vi "Builtins.vi"(6 "args":string[](array[string]), 7 "QD Plugins Dir":path, 8 "error in (no error)":errorcluster, 9 "Shift?":bool, 10 "Focus":enum8{"FP", "BD"}(ring), 11 "VI Refnum":refnum<vi>) -> (0 "error out":errorcluster)   [LabVIEW 2019]
doc: "Built-in script shortcuts\n\nUsage: Ctrl-Space + \"<shortcut>\" + Ctrl-S\n\nCreated by: Ryan Pacini\n\n[SCRIPT]\n--=Rename Label\n--c=Rename Caption\n--iconlib=Edit Library Icon\n0=Open in File Explore\na=Arrange\naa=Align Left Edges\nad=Align Right Edges\nah=Align Horizontal Centers\nas=Align Bottom Edges\nav=Align Vertical Centers\naw=Align Top Edges\nc=Connect Pane\ncf=Cluster Size Fit\nch=Cluster Size Horizontally\ncn=Cluster Size None\ncv=Cluster Size Vertically\nd=Distribute Vertical Compress\nda=Distribute Left Edges\ndd=Distribute Right Edges\ndf=Distribute Horizontal Compress \ndh=Distribute Horizontal Centers\ndhg=Distribute Horizontal Gap\nds=Distribute Bottom Edges\ndv=Distribute Vertical Centers\ndvg=Distribute Vertical Gap\ndw=Distribute Top Edges\ne=Resizes Window\ner=Error Structure\nhb=Hide Inc/Dec Buttons\nhc=Hide Caption\nhi=Hide Index Display\nhl=Hide Label\nhr=Hide Radix\nhs=Hide Scrollbars\nm=Merge Icon Layers\no=Reset Panel Origins\nrb=Radix Binary or Backslash\nrd=Radix Decimal or Normal\nrx=Radix Hex\nsb=Show Inc/Dec Buttons\nsc=Show Caption\nsi=Show Index Display\nsl=Show Label\nss=Show Scrollbars\nsel=Select Controls and Indicators\nselc=Select Controls\nseli=Select Indicators\nseln=Select None\nsg=Snap to Panel Grid\nu8=Change to U8\nu16=Change to U16\nu32=Change to U32\nu64=Change to U64\ni8=Change to I8\ni16=Change to I16\ni32=Change to I32\ni64=Change to I64\nsgl=Change to SGL\ndbl=Change to DBL\next=Change to EXT\ncsg=Change to CSG\ncdb=Change to CDB\ncxt=Change to CXT"
uses:
  _Builtins/Align.ctl
  _Builtins/Distribute.ctl
  _Builtins/Selection.ctl
  _Builtins/Builtins.lvlib
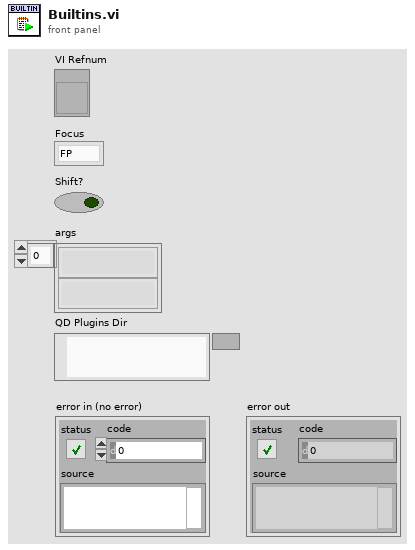
[diagram p1: front panel]
types:
  T1 = typedef "Builtins.lvlib/Align.ctl" = enum8{"Top Edges", "Vertical Centers", "Bottom Edges", "Left Edges", "Horizontal Centers", "Right Edges"}
  T2 = enum32{"Extended Precision", "Double Precision", "Single Precision", "Long", "Word", "Byte", "Unsigned Long", "Unsigned Word", "Unsigned Byte", "Complex Extended", "Complex Double", "Complex Single", "Quad", "Unsigned Quad", "Fixed-Point"}
  T3 = enum8{"None", "SizeToFit", "Horizontally", "Vertically"}
  T4 = typedef "Builtins.lvlib/Distribute.ctl" = enum8{"Top Edges", "Vertical Centers", "Bottom Edges", "Vertical Gap", "Vertical Compress", "Left Edges", "Horizontal Centers", "Right Edges", "Horizontal Gap", "Horizontal Compress"}
  T5 = typedef "Builtins.lvlib/Selection.ctl" = enum8{"None", "Controls", "Indicators", "Both"}
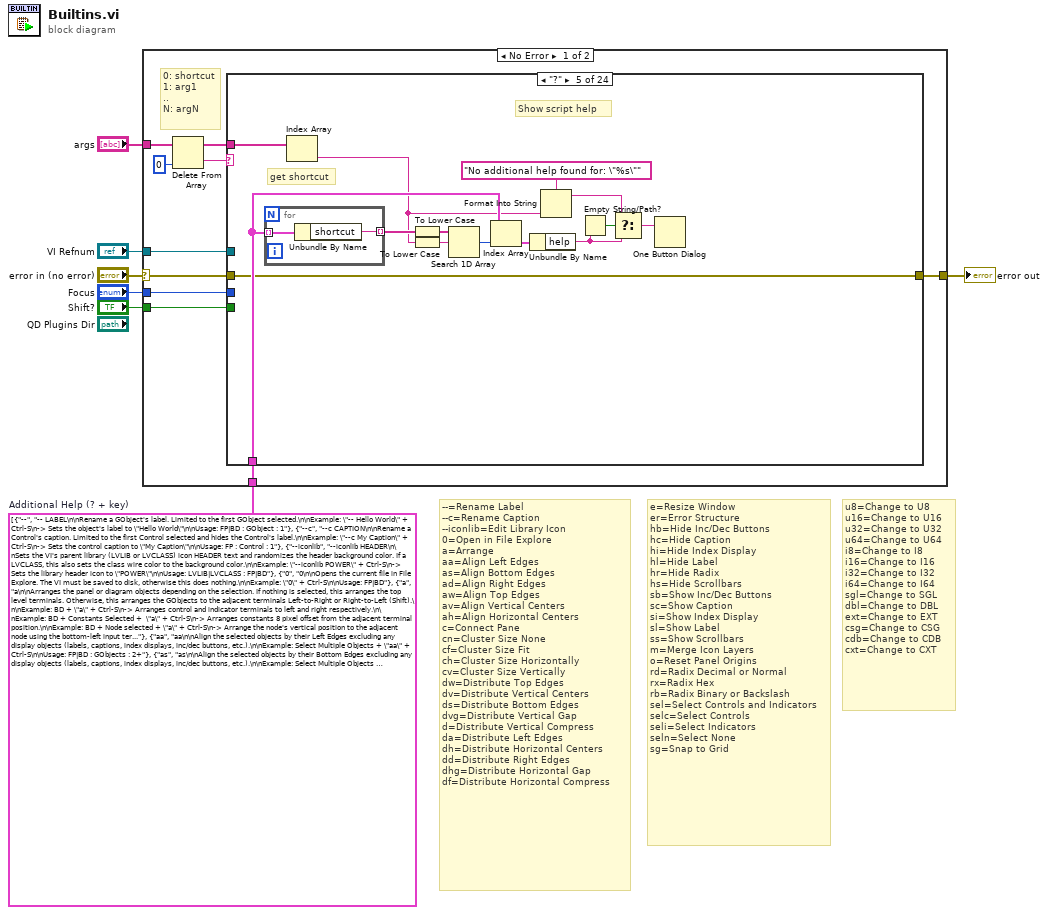
[diagram p0: block diagram]
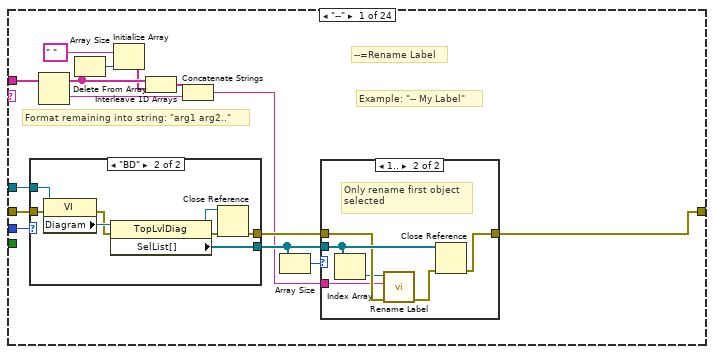
[diagram p2: hidden frame]
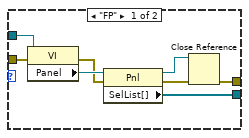
[diagram p3: hidden frame]
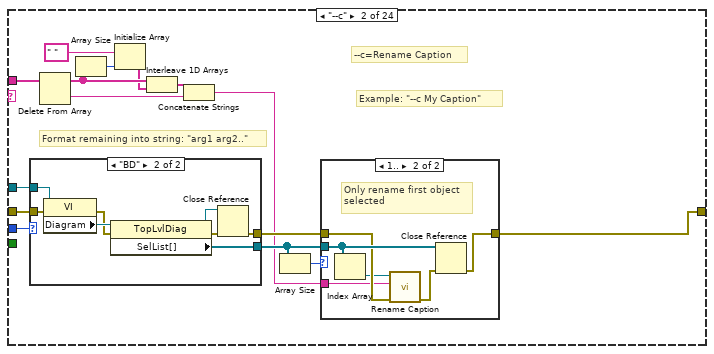
[diagram p5: hidden frame]
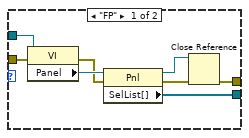
[diagram p6: hidden frame]
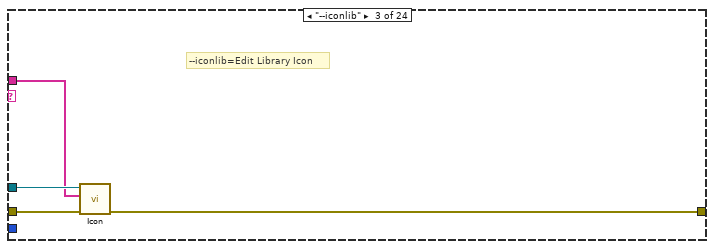
[diagram p8: hidden frame]
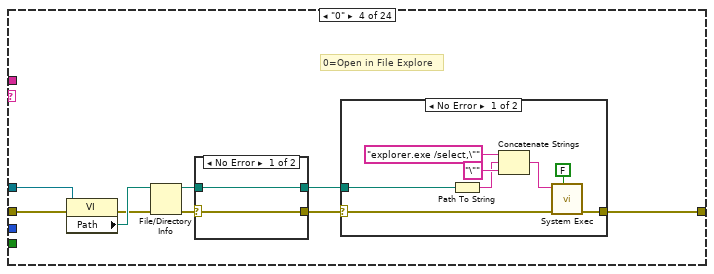
[diagram p9: hidden frame]
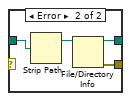
[diagram p10: hidden frame]
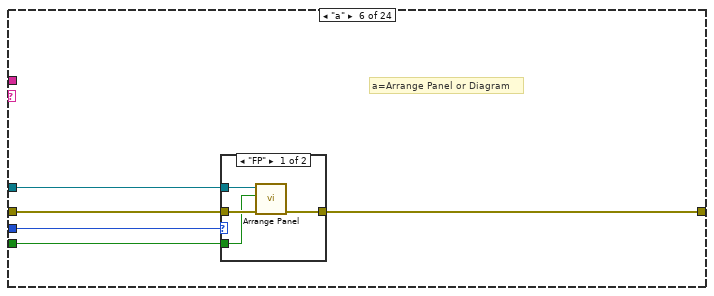
[diagram p12: hidden frame]
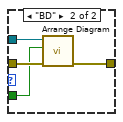
[diagram p13: hidden frame]
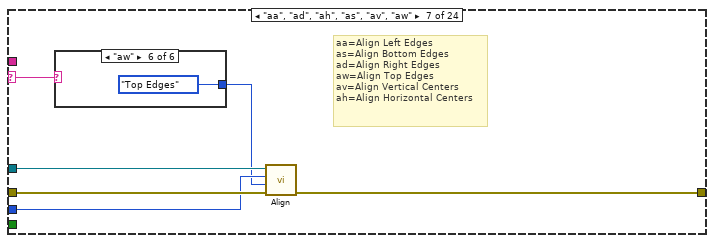
[diagram p14: hidden frame]
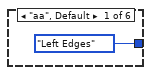
[diagram p15: hidden frame]
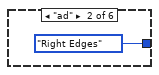
[diagram p16: hidden frame]
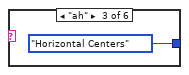
[diagram p17: hidden frame]
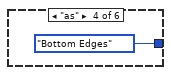
[diagram p18: hidden frame]
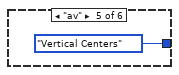
[diagram p19: hidden frame]
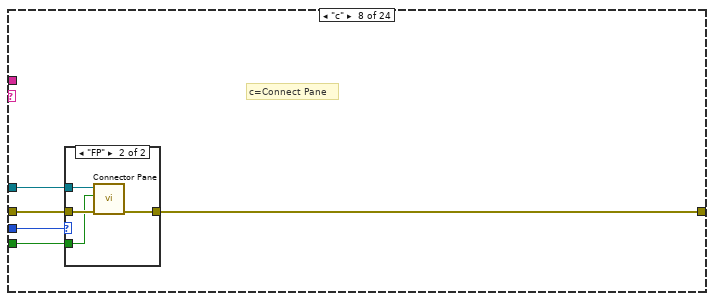
[diagram p20: hidden frame]
diagram:
  w1 = cluster{"shortcut":string, "help":string}[] [{"shortcut"="--", "help"="-- LABEL\n\nRename a GObject's label. Limited to the first GObject selected.\n\nExample: \"-- Hello World\" + Ctrl-S\n-> Sets the object's label to \"Hello World\"\n\nUsage: FP|BD : GObject : 1"}, {"shortcut"="--c", "help"="--c CAPTION\n\nRename a Control's caption. Limited to the first Control selected and hides the Control's label.\n\nExample: \"--c My Caption\" + Ctrl-S\n-> Sets the control caption to \"My Caption\"\n\nUsage: FP : Control : 1"}, {"shortcut"="--iconlib", "help"="--iconlib HEADER\n\nSets the VI's parent library (LVLIB or LVCLASS) icon HEADER text and randomizes the header background color. If a LVCLASS, this also sets the class wire color to the background color.\n\nExample: \"--iconlib POWER\" + Ctrl-S\n-> Sets the library header icon to \"POWER\"\n\nUsage: LVLIB|LVCLASS : FP|BD"}, {"shortcut"="0", "help"="0\n\nOpens the current file in File Explore. The VI must be saved to disk, otherwise this does nothing.\n\nExample: \"0\" + Ctrl-S\n\nUsage: FP|BD"}, {"shortcut"="a", "help"="a\n\nArranges the panel or diagram objects depending on the selection. If nothing is selected, this arranges the top level terminals. Otherwise, this arranges the GObjects to the adjacent terminals Left-to-Right or Right-to-Left (Shift).\n\nExample: BD + \"a\" + Ctrl-S\n-> Arranges control and indicator terminals to left and right respectively.\n\nExample: BD + Constants Selected +  \"a\" + Ctrl-S\n-> Arranges constants 8 pixel offset from the adjacent terminal position.\n\nExample: BD + Node selected + \"a\" + Ctrl-S\n-> Arrange the node's vertical position to the adjacent node using the bottom-left input terminal.\n\nExample: BD + Node selected + \"a\" + Ctrl-Shift-S\n-> Arrange the node's vertical position to the adjacent node using the bottom-right output terminal.\n\nUsage: FP|BD : GObjects : 0+"}, {"shortcut"="aa", "help"="aa\n\nAlign the selected objects by their Left Edges excluding any display objects (labels, captions, index displays, inc/dec buttons, etc.).\n\nExample: Select Multiple Objects + \"aa\" + Ctrl-S\n\nUsage: FP|BD : GObjects : 2+"}, {"shortcut"="as", "help"="as\n\nAlign the selected objects by their Bottom Edges excluding any display objects (labels, captions, index displays, inc/dec buttons, etc.).\n\nExample: Select Multiple Objects + \"as\" + Ctrl-S\n\nUsage: FP|BD : GObjects : 2+"}, {"shortcut"="ad", "help"="ad\n\nAlign the selected objects by their Right Edges excluding any display objects (labels, captions, index displays, inc/dec buttons, etc.).\n\nExample: Select Multiple Objects + \"ad\" + Ctrl-S\n\nUsage: FP|BD : GObjects : 2+"}, {"shortcut"="aw", "help"="aw\n\nAlign the selected objects by their Top Edges excluding any display objects (labels, captions, index displays, inc/dec buttons, etc.).\n\nExample: Select Multiple Objects + \"aw\" + Ctrl-S\n\nUsage: FP|BD : GObjects : 2+"}, {"shortcut"="av", "help"="av\n\nAlign the selected objects by their Vertical Centers excluding any display objects (labels, captions, index displays, inc/dec buttons, etc.).\n\nExample: Select Multiple Objects + \"av\" + Ctrl-S\n\nUsage: FP|BD : GObjects : 2+"}, {"shortcut"="ah", "help"="ah\n\nAlign the selected objects by their Horizontal Centers excluding any display objects (labels, captions, index displays, inc/dec buttons, etc.).\n\nExample: Select Multiple Objects + \"ah\" + Ctrl-S\n\nUsage: FP|BD : GObjects : 2+"}, {"shortcut"="c", "help"="c\n\nWire the Front Panel Controls to the VI Conntector Pane in order of position (top-left to bottom-right). If nothing is selected all unwired controls are connected. Error clusters are wired to the bottom-left and bottom-right terminal. Hold Shift to start wiring by inner columns. Wired terminals are skipped.\n\nExample: FP + \"c\" + Ctrl-S\n-> Wire all controls to VI Connector Pane.\n\nExample: FP + Select Control + \"c\" + Ctrl-Shift-S\n-> Wire selected control to VI Connecto Pane starting with inner column.\n\nUsage: FP : Controls : 0+"}, {"shortcut"="cn", "help"="cn\n\nAutosize the Cluster to None.\n\nExample: Select Cluster + \"cn\" + Ctrl-S\n\nUsage: FP|BD : Cluster : 1+"}, {"shortcut"="cv", "help"="cv\n\nAutosize the Cluster Vertically.\n\nExample: Select Cluster + \"cv\" + Ctrl-S\n\nUsage: FP|BD : Cluster : 1+"}, {"shortcut"="ch", "help"="ch\n\nAutosize the Cluster Horizontally.\n\nExample: Select Cluster + \"ch\" + Ctrl-S\n\nUsage: FP|BD : Cluster : 1+"}, {"shortcut"="cf", "help"="cf\n\nAutosize the Cluster to Fit.\n\nExample: Select Cluster + \"cf\" + Ctrl-S\n\nUsage: FP|BD : Cluster : 1+"}, {"shortcut"="dw", "help"="dw\n\nDistibute the selected objects by their Top Edges including any display objects (labels, captions, index display, inc/dec buttons, etc.).\n\nExample: Select Multiple Objects + \"dw\" + Ctrl-S\n\nUsage: FP|BD : GObjects : 2+"}, {"shortcut"="dv", "help"="dv\n\nDistibute the selected objects by their Vertical Centers including any display objects (labels, captions, index display, inc/dec buttons, etc.).\n\nExample: Select Multiple Objects + \"dv\" + Ctrl-S\n\nUsage: FP|BD : GObjects : 2+"}, {"shortcut"="ds", "help"="ds\n\nDistibute the selected objects by their Bottom Edges including any display objects (labels, captions, index display, inc/dec buttons, etc.).\n\nExample: Select Multiple Objects + \"ds\" + Ctrl-S\n\nUsage: FP|BD : GObjects : 2+"}, {"shortcut"="dvg", "help"="dvg\n\nDistibute the selected objects by their Vertical Gap including any display objects (labels, captions, index display, inc/dec buttons, etc.).\n\nExample: Select Multiple Objects + \"dvg\" + Ctrl-S\n\nUsage: FP|BD : GObjects : 2+"}, {"shortcut"="d", "help"="d\n\nDistibute the selected objects by their Vertical Compress including any display objects (labels, captions, index display, inc/dec buttons, etc.).\n\nExample: Select Multiple Objects + \"d\" + Ctrl-S\n\nUsage: FP|BD : GObjects : 2+"}, {"shortcut"="da", "help"="da\n\nDistibute the selected objects by their Left Edges including any display objects (labels, captions, index display, inc/dec buttons, etc.).\n\nExample: Select Multiple Objects + \"da\" + Ctrl-S"}, {"shortcut"="dh", "help"="dh\n\nDistibute the selected objects by their Horizontal Centers including any display objects (labels, captions, index display, inc/dec buttons, etc.).\n\nExample: Select Multiple Objects + \"dh\" + Ctrl-S\n\nUsage: FP|BD : GObjects : 2+"}, {"shortcut"="dd", "help"="dd\n\nDistibute the selected objects by their Right Edges including any display objects (labels, captions, index display, inc/dec buttons, etc.).\n\nExample: Select Multiple Objects + \"dd\" + Ctrl-S\n\nUsage: FP|BD : GObjects : 2+"}, {"shortcut"="dhg", "help"="dhg\n\nDistibute the selected objects by their Horizontal Gap including any display objects (labels, captions, index display, inc/dec buttons, etc.).\n\nExample: Select Multiple Objects + \"dhg\" + Ctrl-S\n\nUsage: FP|BD : GObjects : 2+"}, {"shortcut"="df", "help"="df\n\nDistibute the selected objects by their Horizontal Compress including any display objects (labels, captions, index display, inc/dec buttons, etc.).\n\nExample: Select Multiple Objects + \"df\" + Ctrl-S\n\nUsage: FP|BD : GObjects : 2+"}, {"shortcut"="e", "help"="e\n\nResize the panel or diagram window to content. This resets the front panel origins to zero.\n\nExample: BD + \"e\" + Ctrl-S\n-> Resizes the diagram window to content with padding.\n\nExample: FP + \"e\" + Ctrl-S\n-> Resets the panel origins and resizes window to bottom-right padding.\n\nUsage: FP|BD"}, {"shortcut"="er", "help"="er\n\nOn the diagram, this wires the selected case structure to the error in and error out terminals. If the case structure selector is already wired, this does nothing. On the panel, this replaces the selected controls with the Error In 3D controls. \n\nExample: BD + Case Structure with Error wires + \"er\" + Ctrl-S\n-> Wires the error terminals to case structure.\n\nExample: FP + Select Control + \"er\" + Ctrl-S\n-> Replaces control with Error In 3D ctl.\n\nUsage: BD : Case Structure : 1 | FP : Control : 1"}, {"shortcut"="hb", "help"="hb\n\nHide the selected Control's Increment/Decrement buttons.\n\nExample: Select Numeric Control + \"hb\" + Ctrl-S\n\nUsage: FP : Controls : 1+"}, {"shortcut"="hc", "help"="hc\n\nHide the selected control's Caption.\n\nExample: Select Control + \"hc\" + Ctrl-S\n\nUsage: FP : Controls : 1+"}, {"shortcut"="hi", "help"="hi\n\nHide the selected array object's Index Display.\n\nExample: Select Array + \"hi\" + Ctrl-S\n\nUsage: FP|BD : Array : 1+"}, {"shortcut"="hl", "help"="hl\n\nHide the selected GObject's Label.\n\nExample: Select GObject + \"hl\" + Ctrl-S\n\nUsage: FP|BD : GObjects : 1+"}, {"shortcut"="hr", "help"="hr\n\nHide the selected Numeric or String Radix Display.\n\nExample: Select Object + \"hr\" + Ctrl-S\n\nUsage: FP|BD : Numeric|String | 1+"}, {"shortcut"="hs", "help"="hs\n\nHide the selected String or Container Vertical Scrollbar.\n\nExample: Select String + \"hs\" + Ctrl-S\n\nUsage: FP|BD : String|Container : 1+"}, {"shortcut"="sb", "help"="sb\n\nShow the selected Control's Increment/Decrement Buttons.\n\nExample: Select Numeric Control + \"sb\" + Ctrl-S\n\nUsage: FP : Controls : 1+"}, {"shortcut"="sc", "help"="sc\n\nShow the selected Control's Caption. This uses the controls label if the caption is not defined.\n\nExample: Select Control + \"sc\" + Ctrl-S\n\nUsage: FP : Controls : 1+"}, {"shortcut"="si", "help"="si\n\nShow the selected Array's Index Display.\n\nExample: Select Array + \"si\" + Ctrl-S\n\nUsage: FP|BD : Array : 1+"}, {"shortcut"="sl", "help"="sl\n\nShow the selected GObject's Label.\n\nExample: Select GObject + \"sl\" + Ctrl-S\n\nUsage: FP|BD : GObjects : 1+"}, {"shortcut"="ss", "help"="ss\n\nShow the selected String or Container Vertical Scrollbars.\n\nExample: Select String + \"ss\" + Ctrl-S\n\nUsage: FP|BD : String|Container | 1+"}, {"shortcut"="m", "help"="m\n\nMerge VI Icon Layers to reduce memory and avoid icon template conflicts.\n\nExample: \"m\" + Ctrl-S\n\nUsage: FP|BD"}, {"shortcut"="o", "help"="o\n\nReset all Front Panel Origins to (0, 0).\n\nExample: \"o\" + Ctrl-S\n\nUsage: FP"}, {"shortcut"="rd", "help"="rd\n\nShow the selected Numeric or String Radix in Decimal (or Default Text).\n\nExample: Select Numeric Control + \"rd\" + Ctrl-S\n-> Shows the radix in decimal (%d)\n\nExample: Select String Control + \"rd\" + Ctrl-S\n-> Shows the radix in default text\n\nUsage: FP|BD : Numeric|String : 1+"}, {"shortcut"="rx", "help"="rx\n\nShow the selected Numeric or String Radix in Hex. If a numeric, this will pad the hex with zeros depending on the numeric representation.\n\nExample: Select U16 Numeric Control + \"rx\" + Ctrl-S\n-> Shows the radix in hex (%04x = '0x0000')\n\nExample: Select String Control + \"rx\" + Ctrl-S\n-> Shows the radix in hex text\n\nUsage: FP|BD : Numeric|String : 1+"}, {"shortcut"="rb", "help"="rb\n\nShow the selected Numeric or String Radix in Binary (or Backslash). If a numeric, this will pad the binary with zeros depending on the numeric representation.\n\nExample: Select U8 Numeric Control + \"rb\" + Ctrl-S\n-> Shows the radix in binary (%08b = '0b00000000')\n\nExample: Select String Control + \"rb\" + Ctrl-S\n-> Shows the radix in backslash text\n\nUsage: FP|BD : Numeric|String : 1+"}, {"shortcut"="sel", "help"="sel\n\nSelect all top-level Control and Indicator Terminals. Used to chain multiple scripts together.\n\nExample: FP + \"sel\" + Ctrl-S\n-> Selects all controls and indicators.\n\nExample: BD + \"sel\" + Ctrl-S\n-> Selects all control and indicator terminals on the top-level diagram.\n\nUsage: FP|BD"}, {"shortcut"="selc", "help"="selc\n\nSelect all top-level Control Terminals. Used to chain multiple scripts together.\n\nExample: FP + \"selc\" + Ctrl-S\n-> Selects all controls.\n\nExample: BD + \"selc\" + Ctrl-S\n-> Selects all control terminals on the top-level diagram.\n\nUsage: FP|BD"}, {"shortcut"="seli", "help"="seli\n\nSelect all top-level Indicator Terminals. Used to chain multiple scripts together.\n\nExample: FP + \"seli\" + Ctrl-S\n-> Selects all indicators.\n\nExample: BD + \"seli\" + Ctrl-S\n-> Selects all indicator terminals on the top-level diagram.\n\nUsage: FP|BD"}, {"shortcut"="seln", "help"="seln\n\nDe-select all. Used to chain multiple scripts together.\n\nExample: FP + \"selc\" + Ctrl-S\n-> De-selects all.\n\nExample: BD + \"selc\" + Ctrl-S\n-> De-selects all.\n\nUsage: FP|BD"}, {"shortcut"="sg", "help"="sg\n\nSnap the selected controls to the nearest panel grid position. If nothing is selected, this snaps all controls. Default grid size is 12 px.\n\nExample: FP + \"sg\" + Ctrl-S\n-> Snaps all controls to nearest grid position.\n\nUsage: FP : Controls : 0+"}, {"shortcut"="u8", "help"="u8\n\nChanges the Numeric Representation to U8.\n\nExample: Select Numeric + \"u8\" + Ctrl-S\n\nUsage: FP|BD : Numeric : 1+"}, {"shortcut"="u16", "help"="u16\n\nChanges the Numeric Representation to U16.\n\nExample: Select Numeric + \"u16\" + Ctrl-S\n\nUsage: FP|BD : Numeric : 1+"}, {"shortcut"="u32", "help"="u32\n\nChanges the Numeric Representation to U32.\n\nExample: Select Numeric + \"u32\" + Ctrl-S\n\nUsage: FP|BD : Numeric : 1+"}, {"shortcut"="u64", "help"="u64\n\nChanges the Numeric Representation to U64.\n\nExample: Select Numeric + \"u64\" + Ctrl-S\n\nUsage: FP|BD : Numeric : 1+"}, {"shortcut"="i8", "help"="i8\n\nChanges the Numeric Representation to I8.\n\nExample: Select Numeric + \"i8\" + Ctrl-S\n\nUsage: FP|BD : Numeric : 1+"}, {"shortcut"="i16", "help"="i16\n\nChanges the Numeric Representation to I16.\n\nExample: Select Numeric + \"i16\" + Ctrl-S\n\nUsage: FP|BD : Numeric : 1+"}, {"shortcut"="i32", "help"="i32\n\nChanges the Numeric Representation to I32.\n\nExample: Select Numeric + \"i32\" + Ctrl-S\n\nUsage: FP|BD : Numeric : 1+"}, {"shortcut"="i64", "help"="i64\n\nChanges the Numeric Representation to I64.\n\nExample: Select Numeric + \"i64\" + Ctrl-S\n\nUsage: FP|BD : Numeric : 1+"}, {"shortcut"="sgl", "help"="sgl\n\nChanges the Numeric Representation to SGL.\n\nExample: Select Numeric + \"sgl\" + Ctrl-S\n\nUsage: FP|BD : Numeric : 1+"}, {"shortcut"="dbl", "help"="dbl\n\nChanges the Numeric Representation to DBL.\n\nExample: Select Numeric + \"dbl\" + Ctrl-S\n\nUsage: FP|BD : Numeric : 1+"}, {"shortcut"="ext", "help"="ext\n\nChanges the Numeric Representation to EXT.\n\nExample: Select Numeric + \"ext\" + Ctrl-S\n\nUsage: FP|BD : Numeric : 1+"}, {"shortcut"="csg", "help"="csg\n\nChanges the Numeric Representation to CSG.\n\nExample: Select Numeric + \"csg\" + Ctrl-S\n\nUsage: FP|BD : Numeric : 1+"}, {"shortcut"="cdb", "help"="cdb\n\nChanges the Numeric Representation to CDB.\n\nExample: Select Numeric + \"cdb\" + Ctrl-S\n\nUsage: FP|BD : Numeric : 1+"}, {"shortcut"="cxt", "help"="cxt\n\nChanges the Numeric Representation to CXT.\n\nExample: Select Numeric + \"cxt\" + Ctrl-S\n\nUsage: FP|BD : Numeric : 1+"}]  # Additional Help (? + key)
  # "u8=Change to U8\nu16=Change to U16\nu32=Change to U32\nu64=Change to U64\ni8=Change to I8\ni16=Change to I16\ni32=Change to I32\ni64=Change to I64\nsgl=Change to SGL\ndbl=Change to DBL\next=Change to EXT\ncsg=Change to CSG\ncdb=Change to CDB\ncxt=Change to CXT"
  # "e=Resize Window\ner=Error Structure\nhb=Hide Inc/Dec Buttons\nhc=Hide Caption\nhi=Hide Index Display\nhl=Hide Label\nhr=Hide Radix\nhs=Hide Scrollbars\nsb=Show Inc/Dec Buttons\nsc=Show Caption\nsi=Show Index Display\nsl=Show Label\nss=Show Scrollbars\nm=Merge Icon Layers\no=Reset Panel Origins\nrd=Radix Decimal or Normal\nrx=Radix Hex\nrb=Radix Binary or Backslash\nsel=Select Controls and Indicators\nselc=Select Controls\nseli=Select Indicators\nseln=Select None\nsg=Snap to Grid"
  # "--=Rename Label\n--c=Rename Caption\n--iconlib=Edit Library Icon\n0=Open in File Explore\na=Arrange\naa=Align Left Edges\nas=Align Bottom Edges\nad=Align Right Edges\naw=Align Top Edges\nav=Align Vertical Centers\nah=Align Horizontal Centers\nc=Connect Pane\ncn=Cluster Size None\ncf=Cluster Size Fit\nch=Cluster Size Horizontally\ncv=Cluster Size Vertically\ndw=Distribute Top Edges\ndv=Distribute Vertical Centers\nds=Distribute Bottom Edges\ndvg=Distribute Vertical Gap\nd=Distribute Vertical Compress\nda=Distribute Left Edges\ndh=Distribute Horizontal Centers\ndd=Distribute Right Edges\ndhg=Distribute Horizontal Gap\ndf=Distribute Horizontal Compress"
  n1 = case shown="No Error" "error in (no error)" {
    selector: "error in (no error)" -> [w17 w384]
    tunnel: "VI Refnum" -> [w16 _]
    tunnel: "Focus" -> [w15 _]
    tunnel: "Shift?" -> [w13 _]
    tunnel: "args" -> [w12 _]
    tunnel: [w14 w384] -> w2
    tunnel: w1 -> [w8 _]
    frame No Error {
      # "0: shortcut\n1: arg1\n..\nN: argN"
      n2 = Delete From Array(array=w12, index=0) -> (deleted portion=w11:string, array with subset deleted=w10:string[])  [unwired: 1 in]
      n3 = case shown="\"?\"" w11 {
        selector: w11 -> [_ _ _ _ _ _ w151 _ w177 w231 w241 _ _ w271 w286 w300 w314 w327 w343 _ _ w363 _ w382]
        tunnel: w17 -> [w32 w70 w97 w106 w128 w142 w156 w167 w176 w230 w246 w259 w264 w270 w284 w298 w312 w326 w342 w352 w356 w367 w375 w383]
        tunnel: w16 -> [w31 w69 w96 w105 _ w141 w155 w166 w175 w229 w245 w260 w263 w269 w283 w297 w311 w325 w341 w353 w357 w366 w374 _]
        tunnel: w15 -> [w26 w64 _ _ _ w139 w153 w164 w173 w228 w244 w257 w261 w268 w282 w296 w310 w324 w340 _ w354 w364 w372 _]
        tunnel: [w29 w67 w95 w104 w128 w140 w154 w165 w174 w225 w243 w258 w262 w265 w280 w293 w307 w321 w337 w351 w355 w365 w373 w383] -> w14
        tunnel: w13 -> [_ _ _ _ _ w138 _ w163 _ _ _ _ _ _ _ _ _ _ _ _ _ _ _ _]
        tunnel: w10 -> [w19 w57 w94 _ w133 _ _ _ _ _ _ _ _ _ _ _ _ _ _ _ _ _ _ _]
        tunnel: w8 -> [_ _ _ _ w130 _ _ _ _ _ _ _ _ _ _ _ _ _ _ _ _ _ _ _]
        frame "--" {
          # "Example: \"-- My Label\""
          # "Format remaining into string: \"arg1 arg2..\""
          # "--=Rename Label"
          n4 = case shown="\"BD\"" w26 {
            tunnel: w32 -> [w40 w48]
            tunnel: w31 -> [w39 w47]
            tunnel: [w35 w43] -> w30
            tunnel: [w33 w41] -> w27
            frame "FP" {
              n5 = property class="VI"(reference=w39, error in=w40) -> (error out=w37:errorcluster, "Panel"=w38:refnum<vi>)  [unwired: 1 out]
              n6 = property class="Pnl"(reference=w38, error in=w37) -> (reference out=w36:refnum<vi>, error out=w34:errorcluster, "SelList[]"=w35:refnum<vi>[])
              n7 = Close Reference(reference=w36, error in (no error)=w34) -> (error out=w33:errorcluster)
            }
            frame "BD" {
              n8 = property class="VI"(reference=w47, error in=w48) -> (error out=w45:errorcluster, "Diagram"=w46:refnum<vi>)  [unwired: 1 out]
              n9 = property class="TopLvlDiag"(reference=w46, error in=w45) -> (reference out=w44:refnum<vi>, error out=w42:errorcluster, "SelList[]"=w43:refnum<vi>[])
              n10 = Close Reference(reference=w44, error in (no error)=w42) -> (error out=w41:errorcluster)
            }
          }
          n11 = Delete From Array(array=w19) -> (deleted portion=w20:string, array with subset deleted=w22:string[])  [unwired: 2 in]
          n12 = Array Size(array=w22) -> (size(s)=w24:i32)
          n13 = Initialize Array(" ", w24) -> (w21:string[])
          n14 = Interleave 1D Arrays(w22, w21) -> (w25:string[])
          n15 = Concatenate Strings(w25, w20) -> (w18:string)
          n16 = Array Size(array=w30) -> (size(s)=w28:i32)
          n17 = case shown="1.." w28 {
            tunnel: w27 -> [w49 w53]
            tunnel: w30 -> [_ w55]
            tunnel: w18 -> [_ w50]
            tunnel: [w49 w54] -> w29
            frame ..0 {
              # "Nothing selected"
            }
            frame 1.. {
              # "Only rename first object\nselected"
              n18 = Index Array(array=w55) -> (element=w52:refnum<vi>)  [unwired: 1 in]
              n19 = call "Rename Label.vi"("error in (no error)"=w53, "Label"=w50, "GObject in"=w52) -> ("error out"=w51:errorcluster)  [unwired: 6 in, 2 out]
              n20 = Close Reference(reference=w55, error in (no error)=w51) -> (error out=w54:errorcluster)
            }
          }
        }
        frame "--c" {
          # "Example: \"--c My Caption\""
          # "Format remaining into string: \"arg1 arg2..\""
          # "--c=Rename Caption"
          n21 = case shown="\"BD\"" w64 {
            tunnel: w70 -> [w78 w86]
            tunnel: w69 -> [w77 w85]
            tunnel: [w73 w81] -> w68
            tunnel: [w71 w79] -> w65
            frame "FP" {
              n22 = property class="VI"(reference=w77, error in=w78) -> (error out=w75:errorcluster, "Panel"=w76:refnum<vi>)  [unwired: 1 out]
              n23 = property class="Pnl"(reference=w76, error in=w75) -> (reference out=w74:refnum<vi>, error out=w72:errorcluster, "SelList[]"=w73:refnum<vi>[])
              n24 = Close Reference(reference=w74, error in (no error)=w72) -> (error out=w71:errorcluster)
            }
            frame "BD" {
              n25 = property class="VI"(reference=w85, error in=w86) -> (error out=w83:errorcluster, "Diagram"=w84:refnum<vi>)  [unwired: 1 out]
              n26 = property class="TopLvlDiag"(reference=w84, error in=w83) -> (reference out=w82:refnum<vi>, error out=w80:errorcluster, "SelList[]"=w81:refnum<vi>[])
              n27 = Close Reference(reference=w82, error in (no error)=w80) -> (error out=w79:errorcluster)
            }
          }
          n28 = Delete From Array(array=w57) -> (deleted portion=w58:string, array with subset deleted=w60:string[])  [unwired: 2 in]
          n29 = Array Size(array=w60) -> (size(s)=w62:i32)
          n30 = Initialize Array(" ", w62) -> (w59:string[])
          n31 = Interleave 1D Arrays(w60, w59) -> (w63:string[])
          n32 = Concatenate Strings(w63, w58) -> (w56:string)
          n33 = Array Size(array=w68) -> (size(s)=w66:i32)
          n34 = case shown="1.." w66 {
            tunnel: w65 -> [w87 w91]
            tunnel: w68 -> [_ w93]
            tunnel: w56 -> [_ w89]
            tunnel: [w87 w92] -> w67
            frame ..0 {
              # "Nothing selected"
            }
            frame 1.. {
              # "Only rename first object\nselected"
              n35 = Index Array(array=w93) -> (element=w90:refnum<vi>)  [unwired: 1 in]
              n36 = call "Rename Caption.vi"("error in (no error)"=w91, "Caption"=w89, "GObject in"=w90) -> ("error out"=w88:errorcluster)  [unwired: 6 in, 2 out]
              n37 = Close Reference(reference=w93, error in (no error)=w88) -> (error out=w92:errorcluster)
            }
          }
        }
        frame "--iconlib" {
          # "--iconlib=Edit Library Icon"
          n38 = call "Icon.vi"("error in (no error)"=w97, "Args"=w94, "VI Refnum in"=w96) -> ("error out"=w95:errorcluster)  [unwired: 7 in, 1 out]
        }
        frame "0" {
          # "0=Open in File Explore"
          n39 = property class="VI"(reference=w105, error in=w106) -> (error out=w98:errorcluster, "Path"=w103:path)  [unwired: 1 out]
          n40 = File/Directory Info(path=w103, error in=w98) -> (path out=w102:path, error out=w100:errorcluster)  [unwired: 5 out]
          n41 = case shown="No Error" w100 {
            selector: w100 -> [w107 _]
            tunnel: w102 -> [w108 w112]
            tunnel: [w107 w110] -> w101
            tunnel: [w108 w109] -> w99
            frame No Error {
            }
            frame Error {
              n42 = Strip Path(path=w112) -> (stripped path=w111:path)  [unwired: 1 out]
              n43 = File/Directory Info(path=w111) -> (path out=w109:path, error out=w110:errorcluster)  [unwired: 1 in, 5 out]
            }
          }
          n44 = case shown="No Error" w101 {
            selector: w101 -> [w113 w121]
            tunnel: [w115 w121] -> w104
            tunnel: w99 -> [w114 _]
            frame No Error {
              n45 = Path To String(path=w114) -> (string=w116:string)
              n46 = Concatenate Strings("explorer.exe /select,\"" ("string"), w116, "\"" ("string")) -> (w118:string)
              n47 = call <vilib>:"System Exec.vi"("wait until completion? (T)"=FALSE, "error in (no error)"=w113, "command line"=w118) -> ("error out"=w115:errorcluster)  [unwired: 5 in, 3 out]
            }
            frame Error {
            }
          }
        }
        frame "?" {
          # "Show script help"
          # "get shortcut"
          n48 = for {
            tunnel: w130 -> [w137] mode=indexing
            tunnel: [w136] -> w135 mode=indexing
            n49 = Unbundle By Name(w137) -> ("shortcut"=w136:string)
          }
          n50 = Index Array(array=w133) -> (element=w124:string)  [unwired: 1 in]
          n51 = To Lower Case(string=w135) -> (all lower case string=w134:string[])
          n52 = To Lower Case(string=w124) -> (all lower case string=w132:string)
          n53 = Search 1D Array(1D array=w134, element=w132) -> (index of element=w131:i32)  [unwired: 1 in]
          n54 = Index Array(array=w130, index=w131) -> (element=w129:cluster{"shortcut":string, "help":string})
          n55 = Unbundle By Name(w129) -> ("help"=w126:string)
          n56 = Format Into String(format string="No additional help found for: \"%s\"", w124) -> (resulting string=w122:string)  [unwired: 2 in, 1 out]
          n57 = Empty String/Path?(string/path=w126) -> (empty?=w127:bool)
          n58 = Select(t=w122, s=w127, f=w126) -> (s? t:f=w125:string)
          n59 = One Button Dialog(message=w125) -> ()  [unwired: 1 in, 1 out]
        }
        frame "a" {
          # "a=Arrange Panel or Diagram"
          n60 = case shown="\"FP\"" w139 {
            tunnel: w142 -> [w146 w150]
            tunnel: w141 -> [w145 w149]
            tunnel: w138 -> [w144 w148]
            tunnel: [w143 w147] -> w140
            frame "FP" {
              n61 = call "Arrange Panel.vi"("error in (no error)"=w146, "Shift?"=w144, "VI Refnum in"=w145) -> ("error out"=w143:errorcluster)  [unwired: 7 in, 1 out]
            }
            frame "BD" {
              n62 = call "Arrange Diagram.vi"("error in (no error)"=w150, "Shift?"=w148, "VI Refnum in"=w149) -> ("error out"=w147:errorcluster)  [unwired: 7 in, 1 out]
            }
          }
        }
        frame "aa", "ad", "ah", "as", "av", "aw" {
          # "aa=Align Left Edges\nas=Align Bottom Edges\nad=Align Right Edges\naw=Align Top Edges\nav=Align Vertical Centers\nah=Align Horizontal Centers"
          n63 = case shown="\"aw\"" w151 {
            tunnel: [Align."Left Edges" ("Align Type") Align."Right Edges" ("Align Type") Align."Horizontal Centers" ("Align Type") Align."Bottom Edges" ("Align Type") Align."Vertical Centers" ("Align Type") Align."Top Edges" ("Align Type")] -> w152
            frame "aa", Default {
            }
            frame "ad" {
            }
            frame "ah" {
            }
            frame "as" {
            }
            frame "av" {
            }
            frame "aw" {
            }
          }
          n64 = call "Align.vi"("error in (no error)"=w156, "Align Type"=w152, "Panel"=w153, "VI Refnum in"=w155) -> ("error out"=w154:errorcluster)  [unwired: 6 in, 1 out]
        }
        frame "c" {
          # "c=Connect Pane"
          n65 = case shown="\"FP\"" w164 {
            tunnel: w167 -> [w168 w172]
            tunnel: w166 -> [_ w171]
            tunnel: [w168 w170] -> w165
            tunnel: w163 -> [_ w169]
            frame "BD" {
            }
            frame "FP" {
              n66 = call "Connector Pane.vi"("error in (no error)"=w172, "Wire Middle? (F)"=w169, "VI Refnum in"=w171) -> ("error out"=w170:errorcluster)  [unwired: 7 in, 1 out]
            }
          }
        }
        frame "cdb", "csg", "cxt", "dbl", "ext", "i16", "i32", "i64", "i8", "sgl", "u16", "u32", "u64", "u8" {
          # "**WARNING: Changing Representation clears the panel/diagram Selection List (LV2019 bug)"
          # "sgl=Change to SGL\ndbl=Change to DBL\next=Change to EXT\ncsg=Change to CSG\ncdb=Change to CDB\ncxt=Change to CXT"
          # "u8=Change to U8\nu16=Change to U16\nu32=Change to U32\nu64=Change to U64\ni8=Change to I8\ni16=Change to I16\ni32=Change to I32\ni64=Change to I64"
          n67 = case shown="\"i16\"" w177 {
            tunnel: [T2."Unsigned Byte" ("Representation") T2."Unsigned Word" ("Representation") T2."Unsigned Long" ("Representation") T2."Unsigned Quad" ("Representation") T2."Byte" ("Representation") T2."Word" ("Representation") T2."Long" ("Representation") T2."Quad" ("Representation") T2."Single Precision" ("Representation") T2."Double Precision" ("Representation") T2."Extended Precision" ("Representation") T2."Complex Single" ("Representation") T2."Complex Double" ("Representation") T2."Complex Extended" ("Representation")] -> w178
            frame "u8", Default {
            }
            frame "u16" {
            }
            frame "u32" {
            }
            frame "u64" {
            }
            frame "i8" {
            }
            frame "i16" {
            }
            frame "i32" {
            }
            frame "i64" {
            }
            frame "sgl" {
            }
            frame "dbl" {
            }
            frame "ext" {
            }
            frame "csg" {
            }
            frame "cdb" {
            }
            frame "cxt" {
            }
          }
          n68 = case shown="\"BD\"" w173 {
            tunnel: w178 -> [w190 w206]
            tunnel: w176 -> [w187 w203]
            tunnel: w175 -> [w186 w202]
            tunnel: [w180 w196] -> w174
            frame "BD" {
              n69 = property class="VI"(reference=w186, error in=w187) -> (error out=w188:errorcluster, "Diagram"=w189:refnum<vi>)  [unwired: 1 out]
              n70 = property class="TopLvlDiag"(reference=w189, error in=w188) -> (reference out=w184:refnum<vi>, error out=w185:errorcluster, "SelList[]"=w183:refnum<vi>[])
              n71 = for {
                tunnel: w183 -> [w194] mode=indexing
                tunnel: w190 -> [w193]
                shift-right: [w191] -> w182
                shift-left: w185 -> [w192]
                n72 = call "Numeric Representation.vi"("error in (no error)"=w192, "Representation"=w193, "GObject in"=w194) -> ("error out"=w191:errorcluster)  [unwired: 6 in, 2 out]
              }
              n73 = invoke class="TopLvlDiag" method="Make Selection"(reference=w184, error in=w182, "Objects"=w183) -> (reference out=w179:refnum<vi>, error out=w181:errorcluster)  [unwired: 1 in, 2 out]
              n74 = Close Reference(reference=w179, error in (no error)=w181) -> (error out=w180:errorcluster)
            }
            frame "FP" {
              n75 = property class="VI"(reference=w202, error in=w203) -> (error out=w204:errorcluster, "Panel"=w205:refnum<vi>)  [unwired: 1 out]
              n76 = property class="Pnl"(reference=w205, error in=w204) -> (reference out=w200:refnum<vi>, error out=w201:errorcluster, "SelList[]"=w199:refnum<vi>[])
              n77 = for {
                tunnel: w199 -> [w210] mode=indexing
                tunnel: w206 -> [w209]
                shift-right: [w207] -> w198
                shift-left: w201 -> [w208]
                n78 = call "Numeric Representation.vi"("error in (no error)"=w208, "Representation"=w209, "GObject in"=w210) -> ("error out"=w207:errorcluster)  [unwired: 6 in, 2 out]
              }
              n79 = invoke class="Pnl" method="Make Selection"(reference=w200, error in=w198, "Objects"=w199) -> (reference out=w195:refnum<vi>, error out=w197:errorcluster)  [unwired: 1 in, 2 out]
              n80 = Close Reference(reference=w195, error in (no error)=w197) -> (error out=w196:errorcluster)
            }
          }
        }
        frame "cf", "ch", "cn", "cv" {
          # "cn=Cluster Size None\ncf=Cluster Size Fit\nch=Cluster Size Horizontally\ncv=Cluster Size Vertically"
          n81 = case shown="\"cf\"" w231 {
            tunnel: [T3."SizeToFit" ("AutoSize") T3."Horizontally" ("AutoSize") T3."None" ("AutoSize") T3."Vertically" ("AutoSize")] -> w232
            frame "cf" {
            }
            frame "ch" {
            }
            frame "cn" {
            }
            frame "cv", Default {
            }
          }
          n82 = call "Selection List.vi"("error in (no error)"=w230, "Focus"=w228, "VI Refnum in"=w229) -> ("error out"=w227:errorcluster, "SelList[]"=w226:refnum<vi>[])  [unwired: 5 in, 2 out]
          n83 = for {
            tunnel: w226 -> [w234] mode=indexing
            tunnel: w232 -> [w233]
            shift-right: [w235] -> w225
            shift-left: w227 -> [w236]
            n84 = call "Cluster Autosize.vi"("error in (no error)"=w236, "AutoSize"=w233, "GObject in"=w234) -> ("error out"=w235:errorcluster)  [unwired: 6 in, 2 out]
          }
        }
        frame "d", "da", "dd", "df", "dh", "dhg", "ds", "dv", "dvg", "dw" {
          # "dw=Distribute Top Edges\ndv=Distribute Vertical Centers\nds=Distribute Bottom Edges\ndvg=Distribute Vertical Gap\nd=Distribute Vertical Compress\nda=Distribute Left Edges\ndh=Distribute Horizontal Centers\ndd=Distribute Right Edges\ndhg=Distribute Horizontal Gap\ndf=Distribute Horizontal Compress"
          n85 = case shown="\"d\", Default" w241 {
            tunnel: [Distribute."Vertical Compress" ("Distribute Type") Distribute."Left Edges" ("Distribute Type") Distribute."Right Edges" ("Distribute Type") Distribute."Horizontal Compress" ("Distribute Type") Distribute."Horizontal Centers" ("Distribute Type") Distribute."Horizontal Gap" ("Distribute Type") Distribute."Bottom Edges" ("Distribute Type") Distribute."Vertical Centers" ("Distribute Type") Distribute."Vertical Gap" ("Distribute Type") Distribute."Top Edges" ("Distribute Type")] -> w242
            frame "d", Default {
            }
            frame "da" {
            }
            frame "dd" {
            }
            frame "df" {
            }
            frame "dh" {
            }
            frame "dhg" {
            }
            frame "ds" {
            }
            frame "dv" {
            }
            frame "dvg" {
            }
            frame "dw" {
            }
          }
          n86 = call "Distribute.vi"("error in (no error)"=w246, "Distribute Type"=w242, "Panel"=w244, "VI Refnum in"=w245) -> ("error out"=w243:errorcluster)  [unwired: 6 in, 1 out]
        }
        frame "e" {
          # "e=Resize Window"
          n87 = call "Resize Window.vi"("error in (no error)"=w259, "Focus"=w257, "VI Refnum in"=w260) -> ("error out"=w258:errorcluster)  [unwired: 7 in, 1 out]
        }
        frame "er" {
          # "er=Error Structure"
          n88 = call "Error Structure.vi"("error in (no error)"=w264, "Focus"=w261, "VI Refnum in"=w263) -> ("error out"=w262:errorcluster)  [unwired: 7 in, 1 out]
        }
        frame "hb", "sb" {
          # "hb=Hide Inc/Dec Buttons\nsb=Show Inc/Dec Buttons"
          n89 = case shown="\"sb\"" w271 {
            tunnel: [enum8{"hide", "show"}."hide" ("inc/dec") enum8{"hide", "show"}."show" ("inc/dec")] -> w272
            frame "hb", Default {
            }
            frame "sb" {
            }
          }
          n90 = call "Selection List.vi"("error in (no error)"=w270, "Focus"=w268, "VI Refnum in"=w269) -> ("error out"=w267:errorcluster, "SelList[]"=w266:refnum<vi>[])  [unwired: 5 in, 2 out]
          n91 = for {
            tunnel: w266 -> [w276] mode=indexing
            tunnel: w272 -> [w273]
            shift-right: [w274] -> w265
            shift-left: w267 -> [w275]
            n92 = call "Visible IncDec.vi"("error in (no error)"=w275, "inc/dec"=w273, "GObject in"=w276) -> ("error out"=w274:errorcluster)  [unwired: 5 in, 3 out]
          }
        }
        frame "hc", "sc" {
          # "hc=Hide Caption\nsc=Show Caption"
          n93 = case shown="\"sc\", Default" w286 {
            tunnel: [enum8{"hide", "show"}."hide" ("label") enum8{"hide", "show"}."show" ("label")] -> w285
            frame "hc" {
            }
            frame "sc", Default {
            }
          }
          n94 = call "Selection List.vi"("error in (no error)"=w284, "Focus"=w282, "VI Refnum in"=w283) -> ("error out"=w281:errorcluster, "SelList[]"=w279:refnum<vi>[])  [unwired: 5 in, 2 out]
          n95 = for {
            tunnel: w279 -> [w290] mode=indexing
            shift-right: [w289] -> w280
            shift-left: w281 -> [w288]
            tunnel: w285 -> [w287]
            n96 = call "Visible Caption.vi"("error in (no error)"=w288, "caption"=w287, "GObject in"=w290) -> ("error out"=w289:errorcluster)  [unwired: 5 in, 3 out]
          }
        }
        frame "hi", "si" {
          # "hi=Hide Index Display\nsi=Show Index Display"
          n97 = case shown="\"si\", Default" w300 {
            tunnel: [enum8{"hide", "show"}."hide" ("label") enum8{"hide", "show"}."show" ("label")] -> w299
            frame "hi" {
            }
            frame "si", Default {
            }
          }
          n98 = call "Selection List.vi"("error in (no error)"=w298, "Focus"=w296, "VI Refnum in"=w297) -> ("error out"=w295:errorcluster, "SelList[]"=w294:refnum<vi>[])  [unwired: 5 in, 2 out]
          n99 = for {
            tunnel: w294 -> [w304] mode=indexing
            shift-right: [w301] -> w293
            shift-left: w295 -> [w302]
            tunnel: w299 -> [w303]
            n100 = call "Visible Index.vi"("error in (no error)"=w302, "index display"=w303, "GObject in"=w304) -> ("error out"=w301:errorcluster)  [unwired: 5 in, 3 out]
          }
        }
        frame "hl", "sl" {
          # "hl=Hide Label\nsl=Show Label"
          n101 = case shown="\"hl\"" w314 {
            tunnel: [enum8{"hide", "show"}."hide" ("label") enum8{"hide", "show"}."show" ("label")] -> w313
            frame "hl" {
            }
            frame "sl", Default {
            }
          }
          n102 = call "Selection List.vi"("error in (no error)"=w312, "Focus"=w310, "VI Refnum in"=w311) -> ("error out"=w309:errorcluster, "SelList[]"=w308:refnum<vi>[])  [unwired: 5 in, 2 out]
          n103 = for {
            tunnel: w308 -> [w318] mode=indexing
            shift-right: [w317] -> w307
            shift-left: w309 -> [w316]
            tunnel: w313 -> [w315]
            n104 = call "Visible Label.vi"("error in (no error)"=w316, "label"=w315, "GObject in"=w318) -> ("error out"=w317:errorcluster)  [unwired: 5 in, 3 out]
          }
        }
        frame "hr", "rb", "rd", "rx" {
          # "hr=Radix Hide\nrd=Radix Decimal or Normal\nrx=Radix Hex\nrb=Radix Binary or Backslash"
          n105 = case shown="\"hr\"" w327 {
            tunnel: [enum8{"hide", "dec", "hex", "bin"}."hide" ("radix") enum8{"hide", "dec", "hex", "bin"}."dec" ("radix") enum8{"hide", "dec", "hex", "bin"}."hex" ("radix") enum8{"hide", "dec", "hex", "bin"}."bin" ("radix")] -> w328
            frame "hr" {
            }
            frame "rd", Default {
            }
            frame "rx" {
            }
            frame "rb" {
            }
          }
          n106 = call "Selection List.vi"("error in (no error)"=w326, "Focus"=w324, "VI Refnum in"=w325) -> ("error out"=w323:errorcluster, "SelList[]"=w322:refnum<vi>[])  [unwired: 5 in, 2 out]
          n107 = for {
            tunnel: w322 -> [w332] mode=indexing
            tunnel: w328 -> [w330]
            shift-right: [w329] -> w321
            shift-left: w323 -> [w331]
            n108 = call "Radix.vi"("error in (no error)"=w331, "radix"=w330, "GObject in"=w332) -> ("error out"=w329:errorcluster)  [unwired: 6 in, 2 out]
          }
        }
        frame "hs", "ss" {
          # "hs=Hide Scrollbars\nss=Show Scrollbars"
          n109 = case shown="\"hs\", Default" w343 {
            tunnel: [enum8{"hide", "show"}."hide" ("inc/dec") enum8{"hide", "show"}."show" ("inc/dec")] -> w344
            frame "hs", Default {
            }
            frame "ss" {
            }
          }
          n110 = call "Selection List.vi"("error in (no error)"=w342, "Focus"=w340, "VI Refnum in"=w341) -> ("error out"=w339:errorcluster, "SelList[]"=w338:refnum<vi>[])  [unwired: 5 in, 2 out]
          n111 = for {
            tunnel: w338 -> [w346] mode=indexing
            tunnel: w344 -> [w345]
            shift-right: [w347] -> w337
            shift-left: w339 -> [w348]
            n112 = call "Visible Scrollbar.vi"("error in (no error)"=w348, "scrollbars"=w345, "GObject in"=w346) -> ("error out"=w347:errorcluster)  [unwired: 5 in, 3 out]
          }
        }
        frame "m" {
          # "m=Merge Icon Layers"
          n113 = call "Icon Merge Layers.vi"("error in (no error)"=w352, "VI Refnum in"=w353) -> ("error out"=w351:errorcluster)  [unwired: 8 in, 1 out]
        }
        frame "o" {
          # "o=Reset Panel Origins"
          n114 = case shown="\"FP\"" w354 {
            tunnel: w357 -> [_ w361]
            tunnel: w356 -> [w358 w360]
            tunnel: [w358 w359] -> w355
            frame "BD" {
            }
            frame "FP" {
              n115 = call "Reset Origins.vi"("error in (no error)"=w360, "VI Refnum in"=w361) -> ("error out"=w359:errorcluster)  [unwired: 8 in, 1 out]
            }
          }
        }
        frame "sel", "selc", "seli", "seln" {
          # "sel=Select Controls and Indicators\nselc=Select Controls\nseli=Select Indicators\nseln=Select None"
          n116 = case shown="\"seln\", Default" w363 {
            tunnel: [Selection."Controls" ("Selection") Selection."None" ("Selection") Selection."Indicators" ("Selection") Selection."Both" ("Selection")] -> w362
            frame "selc" {
            }
            frame "seln", Default {
            }
            frame "seli" {
            }
            frame "sel" {
            }
          }
          n117 = call "Select Controls.vi"("error in (no error)"=w367, "Selection"=w362, "Focus"=w364, "VI Refnum in"=w366) -> ("error out"=w365:errorcluster)  [unwired: 6 in, 1 out]
        }
        frame "sg" {
          # "sg=Snap to Grid"
          n118 = case shown="\"FP\"" w372 {
            tunnel: w375 -> [w376 w377]
            tunnel: w374 -> [_ w378]
            tunnel: [w376 w379] -> w373
            frame "BD" {
            }
            frame "FP" {
              n119 = call "Snap to Grid.vi"("error in (no error)"=w377, "VI Refnum in"=w378) -> ("error out"=w379:errorcluster)  [unwired: 8 in, 1 out]
            }
          }
        }
        frame Default {
          n120 = Format Into String(format string="Script Built-Ins\n\nUnknown shortcut: %s", w382) -> (resulting string=w380:string)  [unwired: 2 in, 1 out]
          n121 = One Button Dialog(message=w380) -> ()  [unwired: 1 in, 1 out]
        }
      }
    }
    frame Error {
    }
  }
  "error out" <- w2
